vi "RB2 Example 2.vi"() -> ()   [LabVIEW 2012]
panel:
  out "Closed":bool
  in  "LED ON":bool
  out "switch state":dbl
  out "Pot Volts":dbl(knob) scale=0.0..5.0 scale format="%_2g"
  in  "Servo Position":i32(slide)=1500 scale=500.0..2500.0
  out "String Received":string
  out "return count":u32
  out "bytes written":u32
  out "Blinky":bool
  in  "String":string="$CS1500L1\n"
  in  "stop":bool
  in  "VISA resource name":refnum<visa-resource-name>="COM7"
  # "This routine sends commands to the Arbotix-M board using an XBEE radio link\nIt sends:\n1. The desired servo position in microseconds\n2. The desired LED state, on or off.\nIt receives:\n3.  The position the the potentiometer in volts\n4.  The state the the manaul switch."
  # "SENT TO ARBOTIX-M"
  # "RECEIVED FROM ABROTIX-M"
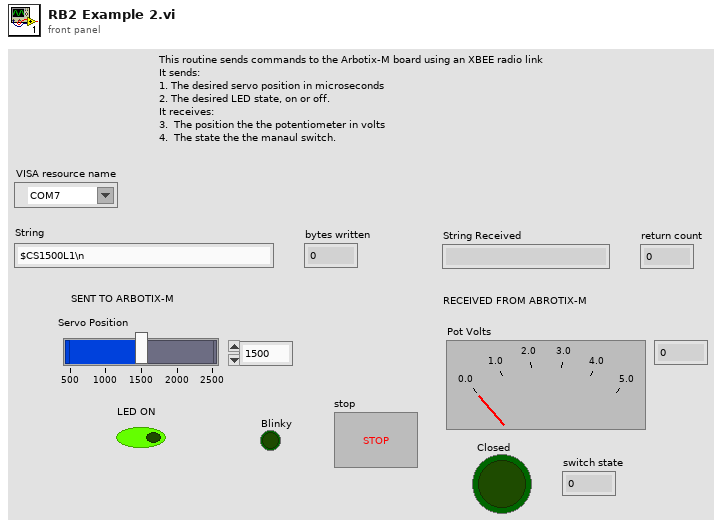
[diagram p1: front panel]
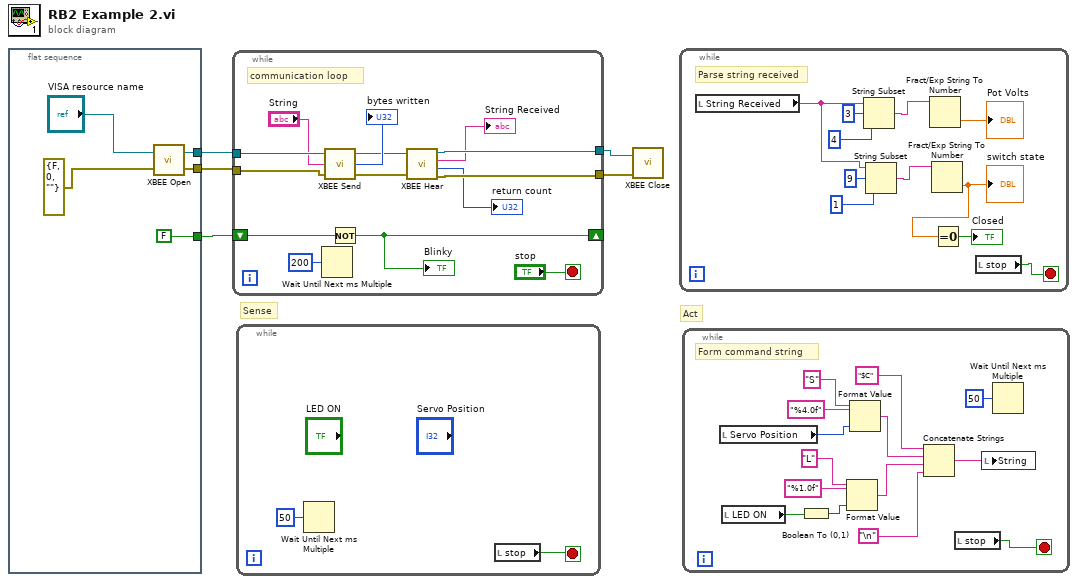
[diagram p0: block diagram]
diagram:
  # "Act"
  # "Sense"
  n1 = flat-sequence {
    tunnel: [w10] -> w5
    tunnel: [w9] -> w4
    tunnel: [FALSE] -> w1
    frame #0 {
      n2 = call "XBEE Open.vi"("error in"=errorcluster {"status"=FALSE, "code"=0, "source"=""}, "VISA resource name"="VISA resource name") -> ("error out"=w9:errorcluster, "VISA resource name out"=w10:refnum<visa-resource-name>)
    }
  }
  n3 = while {
    tunnel: w5 -> [w23]
    tunnel: w4 -> [w22]
    tunnel: [w17] -> w3
    tunnel: [w16] -> w2
    shift-right: [w20] -> _
    shift-left: w1 -> [w21]
    stop <- "stop" stop-if-true
    # "communication loop"
    n4 = Wait Until Next ms Multiple(millisecond multiple=u32 200) -> ()  [unwired: 1 out]
    n5 = call "XBEE Send.vi"("error in (no error)"=w22, "String"="String", "VISA resource name"=w23) -> ("error out"=w13:errorcluster, "return count"=→"bytes written":u32, "VISA resource name out"=w14:refnum<visa-resource-name>)
    n6 = Not(x=w21) -> (.not. x?=w20:bool)
    "Blinky" <- w20
    n7 = call "XBEE Hear.vi"("VISA resource name"=w14, "error in (no error)"=w13) -> ("VISA resource name out"=w17:refnum<visa-resource-name>, "String Received"=→"String Received":string, "return count"=→"return count":u32, "error out"=w16:errorcluster)
  }
  n8 = while {
    stop <- w26 stop-if-true
    n9 = Wait Until Next ms Multiple(millisecond multiple=u32 50) -> ()  [unwired: 1 out]
    n10 = local read "stop"() -> (w26:bool)
  }
  n11 = call "XBEE Close.vi"("error in (no error)"=w2, "VISA resource name"=w3) -> ()
  n12 = while {
    stop <- w35 stop-if-true
    # "Parse string received"
    n13 = local read "String Received"() -> (w29:string)
    n14 = String Subset(string=w29, offset (0)=3, length (rest)=4 ("length (rest)")) -> (substring=w34:string)
    n15 = String Subset(string=w29, offset (0)=9, length (rest)=1 ("length (rest)")) -> (substring=w32:string)
    n16 = Fract/Exp String To Number(string=w34) -> (number=→"Pot Volts":dbl)  [unwired: 3 in, 1 out]
    n17 = Fract/Exp String To Number(string=w32) -> (number=w27:dbl)  [unwired: 3 in, 1 out]
    "switch state" <- w27
    n18 = Equal To 0?(x=w27) -> (x = 0?=→"Closed":bool)
    n19 = local read "stop"() -> (w35:bool)
  }
  n20 = while {
    stop <- w51 stop-if-true
    # "Form command string"
    n21 = local read "Servo Position"() -> (w48:i32)
    n22 = local read "LED ON"() -> (w41:bool)
    n23 = Boolean To (0,1)(Boolean=w41) -> (0, 1=w40:i16)
    n24 = Format Value(string ("")="L", format string="%1.0f", value (0)=w40) -> (output string=w43:string)
    n25 = Format Value(string ("")="S", format string="%4.0f", value (0)=w48) -> (output string=w44:string)
    n26 = Concatenate Strings("$C", w44, w43, "\n") -> (w38:string)
    n27 = local read "stop"() -> (w51:bool)
    n28 = local write "String"(w38) -> ()
    n29 = Wait Until Next ms Multiple(millisecond multiple=u32 50) -> ()  [unwired: 1 out]
  }
